vi "Configure Math (Spectrum).vi"(7 "Operator (1: Subtract)":u16(ring)=1 items=["Add", "Subtract"], 8 "error in (no error)":errorcluster, 9 "2nd RF Source (1: Average)":u16(ring)=1 items=["Normal", "Average", "Maximum Peak Hold", "Minimum Peak Hold"], 10 "1st RF Source (0: Normal)":u16(ring) items=["Normal", "Average", "Maximum Peak Hold", "Minimum Peak Hold"], 11 "VISA resource name":refnum<visa-resource-name>) -> (0 "error out":errorcluster, 3 "VISA resource name out":refnum<visa-resource-name>)   [LabVIEW 2009, in "Tektronix DPO MSO 2000 4000 Series.lvlib"]
doc: "Configures a math channel to perform math operations on RF Channels.\n\n<B>Note:</B>\n This VI applies only to <B>MDO series</B> oscilloscopes"
uses:
  <instrlib>/Tektronix DPO MSO 2000 4000 Series/Tektronix DPO MSO 2000 4000 Series.lvlib
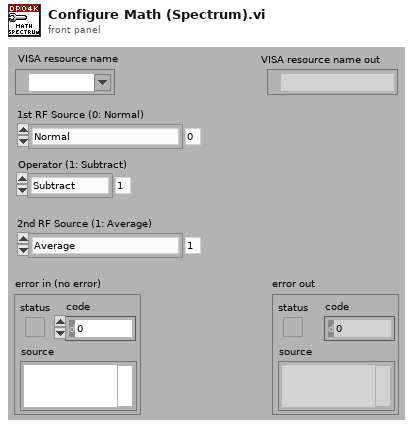
[diagram p1: front panel]
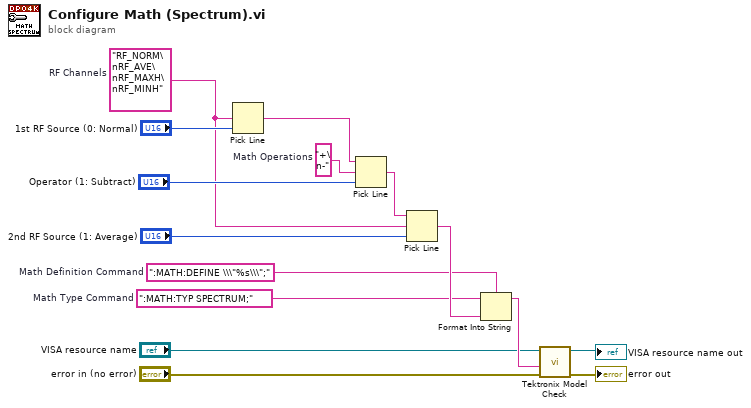
[diagram p0: block diagram]
diagram:
  w6 = ":MATH:DEFINE \\\"%s\\\";"  # Math Definition Command
  w7 = ":MATH:TYP SPECTRUM;"  # Math Type Command
  w14 = "+\n-"  # Math Operations
  w10 = "RF_NORM\nRF_AVE\nRF_MAXH\nRF_MINH"  # RF Channels
  n1 = Pick Line(multi-line string=w10, line index="1st RF Source (0: Normal)") -> (output string=w12:string)  [unwired: 1 in]
  n2 = Pick Line(string ("")=w12, multi-line string=w14, line index="Operator (1: Subtract)") -> (output string=w11:string)
  n3 = Pick Line(string ("")=w11, multi-line string=w10, line index="2nd RF Source (1: Average)") -> (output string=w8:string)
  n4 = Format Into String(format string=w6, initial string=w7, w8) -> (resulting string=w5:string)  [unwired: 1 in, 1 out]
  n5 = call <instrlib>:"Tektronix Model Check.vi"("error in (no error)"="error in (no error)", "Command String"=w5, "VISA resource name"="VISA resource name") -> ("error out"=→"error out":errorcluster, "VISA resource name out"=→"VISA resource name out":refnum<visa-resource-name>)  [unwired: 7 in]
